vi "Willy Wonka.vi"() -> ()   [LabVIEW 2018]
panel:
  out "String 2":string
  out "String":string
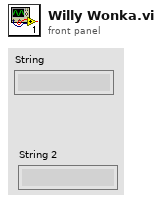
[diagram p1: front panel]
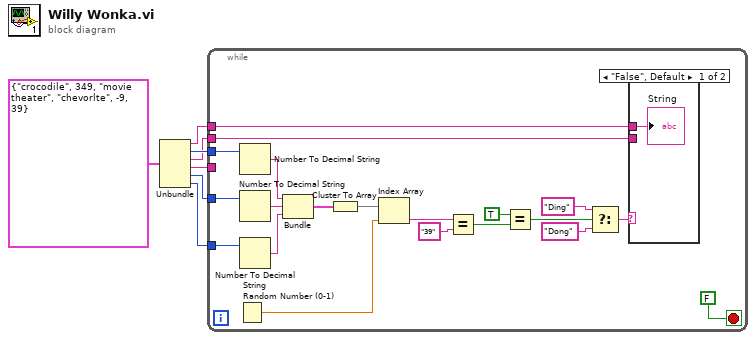
[diagram p0: block diagram]
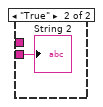
[diagram p2: hidden frame]
diagram:
  n1 = Unbundle(cluster{string, i32, string, string, i32, i32} {"crocodile", 349, "movie theater", "chevorlte", -9, 39}) -> (w3:string, w6:i32, w1:string, w2:string, w5:i32, w4:i32)
  n2 = while {
    tunnel: w6 -> [w26]
    tunnel: w5 -> [w25]
    tunnel: w4 -> [w24]
    tunnel: w3 -> [w10]
    tunnel: w2 -> [_]
    tunnel: w1 -> [w9]
    stop <- FALSE stop-if-true
    n3 = Random Number (0-1)() -> (number: 0 to 1=w8:dbl)
    n4 = Number To Decimal String(number=w26) -> (decimal integer string=w15:string)  [unwired: 1 in]
    n5 = Number To Decimal String(number=w25) -> (decimal integer string=w16:string)  [unwired: 1 in]
    n6 = Number To Decimal String(number=w24) -> (decimal integer string=w14:string)  [unwired: 1 in]
    n7 = Bundle(w15, w16, w14) -> (w17:cluster{string, string, string})  [unwired: 1 in]
    n8 = Cluster To Array(cluster=w17) -> (array=w18:string[])
    n9 = Index Array(array=w18, index=w8) -> (element=w13:string)
    n10 = Equal?(x=w13, y="39") -> (x = y?=w19:bool)
    n11 = Equal?(x=TRUE, y=w19) -> (x = y?=w21:bool)
    n12 = Select(t="Ding", s=w21, f="Dong") -> (s? t:f=w11:string)
    n13 = case shown="\"False\", Default" w11 {
      tunnel: w10 -> [w28 _]
      tunnel: w9 -> [_ w29]
      frame "False", Default {
        "String" <- w28
      }
      frame "True" {
        "String 2" <- w29
      }
    }
  }
